vi "FSC.vi"(0 "System no.":i32=1 min=1 step=1, 1 "Board":i32=1 min=1 max=5 step=1, 2 "Axis 1 to scan":string, 3 "Axis 2 to scan":string, 4 "Range axis 1":dbl=0.1 format="%.4f", 5 "error in":errorcluster, 6 "Treshold level":dbl=0.1 format="%.3f", 7 "Step size":dbl=0.05 format="%.4f", 9 "Range axis 2":dbl=0.1 format="%.4f", 10 "Use #7 polling?":bool, 11 "Timeout (s)":dbl=300.0 min=1.0 max=4.0 step=1.0 format="%.2f", 12 "Stop refnum":refnum<vi>) -> (14 "Scan successful?":bool, 19 "error out":errorcluster)   [LabVIEW 2026]
doc: "Performs a 2D scan in specified axes, waits until scan is ready using #7 polling (if checked) and indicates whether scan was successful or not. If Stop refnum or Local stop is TRUE, VI sends #24 and stops. For a square scan, Range axis 2 must be identical to Range axis 1, otherwise a rectangular scan is performed. Timeout is only valid if Use #7 polling is FALSE.\n\nC-880: Use #7 polling = TRUE\nC-887, F-206, M-8X0: Use #7 polling = FALSE, Range axis 2 must be identical with Range axis 1 (no rectangular scan implemented). For GCS syntax version = GCS 2.0 or higher (check with CSV?.vi. If CSV?.vi is not supported, syntax version is GCS 1.0), VI calls FSS? automatically to determine if scan was successful or not."
uses:
  Communication/Syntax.ctl
  Communication/Global1.vi
panel:
  in  "Local stop":bool
  # "Performs an 2D scan in specified axes, waits until scan is \nready (using #7 polling if checked) and indicates whether scan was\nsuccessful or not.  If Stop refnum or Local stop is TRUE, VI sends #24 \nand stops. For a square scan, \"Range axis 2\" must be identical to \n\"Range axis 1\", otherwise a rectangular scan is performed. \"Timeout\" \nis only valid if \"Use #7 polling\" is FALSE."
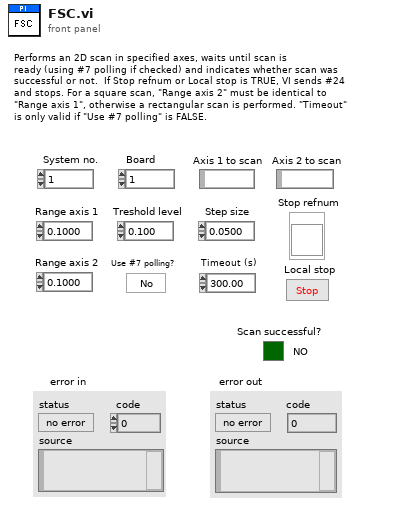
[diagram p1: front panel]
types:
  T1 = typedef "Syntax.ctl" = enum16{"GCS 1.0", "GCS 2.0", "GCS 3.0"}
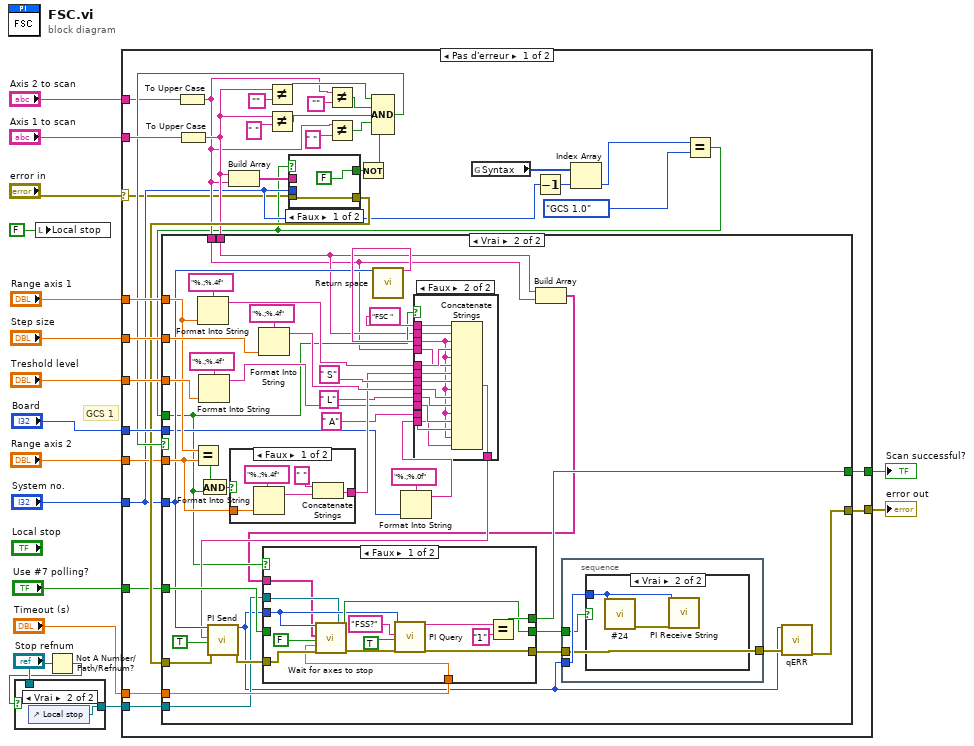
[diagram p0: block diagram]
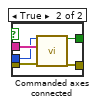
[diagram p3: hidden frame]
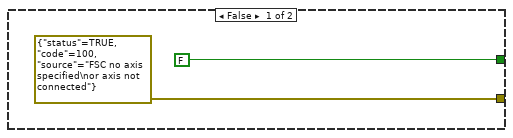
[diagram p4: hidden frame]
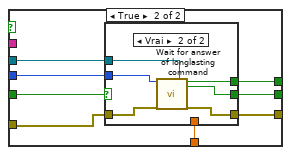
[diagram p5: hidden frame]
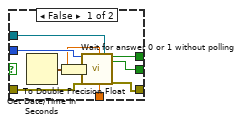
[diagram p6: hidden frame]
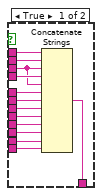
[diagram p7: hidden frame]
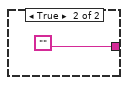
[diagram p9: hidden frame]
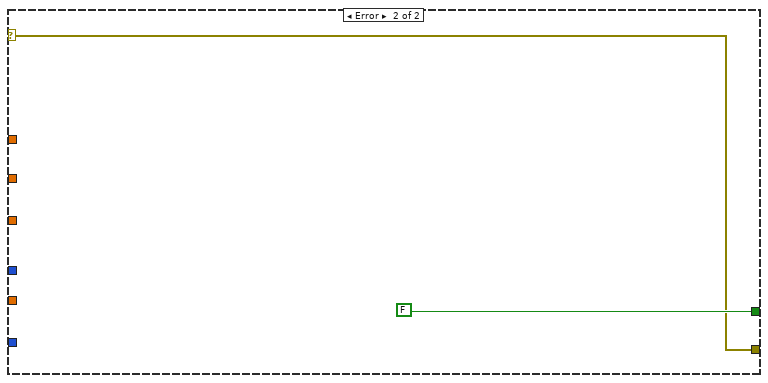
[diagram p10: hidden frame]
diagram:
  # "GCS 1"
  n1 = local write "Local stop"(FALSE ("Local stop")) -> ()
  n2 = Not A Number/Path/Refnum?(number/path/refnum="Stop refnum") -> (NaN/Path/Refnum?=w3:bool)
  n3 = case shown="Vrai" w3 {
    tunnel: [w18 w19] -> w2
    tunnel: "Stop refnum" -> [w18 _]
    frame False {
    }
    frame True {
      n4 = control-ref of="Local stop"() -> (w19:refnum<vi>)
    }
  }
  n5 = case shown="Pas d'erreur" "error in" {
    selector: "error in" -> [w21 w175]
    tunnel: "System no." -> [w23 _]
    tunnel: [w42 w175] -> w16
    tunnel: "Axis 1 to scan" -> [w53 _]
    tunnel: [w41 FALSE] -> w14
    tunnel: "Board" -> [w48 _]
    tunnel: "Range axis 1" -> [w47 _]
    tunnel: "Step size" -> [w46 _]
    tunnel: "Treshold level" -> [w45 _]
    tunnel: "Axis 2 to scan" -> [w37 _]
    tunnel: "Use #7 polling?" -> [w30 _]
    tunnel: "Timeout (s)" -> [w29 _]
    tunnel: "Range axis 2" -> [w28 _]
    tunnel: w2 -> [w27 _]
    frame No Error {
      n6 = To Upper Case(1:w37) -> (0:w31:string)
      n7 = To Upper Case(1:w53) -> (0:w32:string)
      n8 = Build Array(w32, w31) -> (w49:string[])
      n9 = Not Equal?(x=w32, y="") -> (x != y?=w50:bool)
      n10 = Not Equal?(x=w32, y=" ") -> (x != y?=w35:bool)
      n11 = Not Equal?(x=w31, y="") -> (x != y?=w34:bool)
      n12 = Not Equal?(x=w31, y=" ") -> (x != y?=w33:bool)
      n13 = global read "Global1.vi" "Syntax"() -> (w24:T1[])
      n14 = Decrement(x=w23) -> (x-1=w25:i32)
      n15 = Index Array(array=w24, index=w25) -> (element=w26:T1)
      n16 = Equal?(x=w26, y=Syntax."GCS 1.0") -> (x = y?=w22:bool)
      n17 = case shown="Faux" w22 {
        tunnel: w49 -> [_ w60]
        tunnel: w21 -> [w54 w59]
        tunnel: [w54 w58] -> w43
        tunnel: [FALSE ("Controller error") w57] -> w40
        tunnel: w23 -> [_ w56]
        frame False {
        }
        frame True {
          n18 = call "Commanded axes connected.vi"("System no."=w56, "Commanded axes"=w60, "error in"=w59) -> ("Controller error"=w57:bool, "error out"=w58:errorcluster)  [unwired: 15 out]
        }
      }
      n19 = Not(x=w40) -> (.not. x?=w39:bool)
      n20 = Compound Arithmetic op=AND(w50, w34, w35, w33, w39) -> (w44:bool)
      n21 = case shown="Vrai" w44 {
        tunnel: w48 -> [_ w69]
        tunnel: w47 -> [_ w87]
        tunnel: w46 -> [_ w93]
        tunnel: w32 -> [_ w65]
        tunnel: w45 -> [_ w95]
        tunnel: w43 -> [_ w100]
        tunnel: w23 -> [_ w74]
        tunnel: [errorcluster {"status"=TRUE, "code"=100, "source"="FSC no axis specified\nor axis not connected"} ("error out") w81] -> w42
        tunnel: [FALSE w80] -> w41
        tunnel: w31 -> [_ w64]
        tunnel: w30 -> [_ w91]
        tunnel: w29 -> [_ w90]
        tunnel: w28 -> [_ w86]
        tunnel: w27 -> [_ w77]
        tunnel: w22 -> [_ w66]
        frame False {
        }
        frame True {
          n22 = Equal?(x=w87, y=w86) -> (x = y?=w73:bool)
          n23 = Format Into String(format string="%.;%.4f" ("Format String"), w87) -> (resulting string=w92:string)  [unwired: 2 in, 1 out]
          n24 = Format Into String(format string="%.;%.4f" ("Format String"), w95) -> (resulting string=w83:string)  [unwired: 2 in, 1 out]
          n25 = And(x=w73, y=w66) -> (x .and. y?=w72:bool)
          n26 = case shown="Faux" w72 {
            tunnel: w86 -> [w172 _]
            tunnel: [w169 ""] -> w85
            frame False {
              n27 = Format Into String(format string="%.;%.4f" ("Format String"), w172) -> (resulting string=w170:string)  [unwired: 2 in, 1 out]
              n28 = Concatenate Strings(" ", w170) -> (w169:string)
            }
            frame True {
            }
          }
          n29 = Format Into String(format string="%.;%.4f" ("Format String"), w93) -> (resulting string=w89:string)  [unwired: 2 in, 1 out]
          n30 = call "Return space.vi"("System no."=w74) -> ("String out"=w75:string)  [unwired: 1 in, 17 out]
          n31 = Format Into String(format string="%.;%.0f" ("Format String"), w69) -> (resulting string=w68:string)  [unwired: 2 in, 1 out]
          n32 = case shown="Faux" w66 {
            tunnel: [w150 w163] -> w67
            tunnel: w92 -> [w149 w156]
            tunnel: w89 -> [w148 w162]
            tunnel: " S" -> [w147 w161]
            tunnel: w85 -> [w146 w154]
            tunnel: " L" -> [w145 w160]
            tunnel: w83 -> [w144 w159]
            tunnel: "FSC " -> [w143 w158]
            tunnel: w65 -> [w142 w157]
            tunnel: w64 -> [w141 w155]
            tunnel: w75 -> [w140 w151]
            tunnel: " A" -> [w139 w153]
            tunnel: w68 -> [w138 w152]
            frame True {
              n33 = Concatenate Strings(w143, w142, w140, w141, w140, w149, w146, w147, w148, w145, w144, w139, w138) -> (w150:string)
            }
            frame False {
              n34 = Concatenate Strings(w158, w157, w151, w156, w151, w155, w154, w161, w151, w162, w160, w151, w159, w153, w151, w152) -> (w163:string)
            }
          }
          n35 = call "PI Send.vi"("System no."=w74, "String to send"=w67, "Attach termination char.?"=TRUE ("Attach Linefeed?"), "error in"=w100) -> ("error out"=w98:errorcluster)  [unwired: 2 in, 13 out]
          n36 = Build Array(w65, w64) -> (w63:string[])
          n37 = case shown="Faux" w66 {
            tunnel: w98 -> [w109 w122]
            tunnel: w91 -> [_ w121]
            tunnel: w90 -> [w104 w120]
            tunnel: [w108 w119] -> w80
            tunnel: [w102 w118] -> w79
            tunnel: [w107 w117] -> w78
            tunnel: w77 -> [w105 w116]
            tunnel: w74 -> [w106 w115]
            tunnel: w63 -> [w103 _]
            frame False {
              n38 = call "Wait for axes to stop.vi"("System no."=w106, "Axes to wait for"=w103, "With status bit polling?"=FALSE, "Timeout (s)"=w104, "error in"=w109, "Stop refnum"=w105) -> ("Stopped"=w107:bool, "error out"=w111:errorcluster)  [unwired: 1 in, 11 out]
              n39 = call "PI Query.vi"("System no."=w106, "String to send"="FSS?", "Attach termination char.?"=TRUE ("Attach Linefeed?"), "error in"=w111) -> ("String read"=w101:string, "error out"=w102:errorcluster)  [unwired: 3 in, 11 out]
              n40 = Equal?(x=w101, y="1") -> (x = y?=w108:bool)
            }
            frame True {
              n41 = case shown="Vrai" w121 {
                tunnel: w115 -> [w131 w137]
                tunnel: w122 -> [w130 w136]
                tunnel: [w129 w135] -> w118
                tunnel: [w128 w134] -> w119
                tunnel: w120 -> [w126 _]
                tunnel: [w124 w133] -> w117
                tunnel: w116 -> [w125 w132]
                frame False {
                  n42 = Get Date/Time In Seconds() -> (seconds since 1Jan1904=w123:timestamp)
                  n43 = To Double Precision Float(number=w123) -> (double precision float=w127:dbl)
                  n44 = call "Wait for answer 0 or 1 without polling.vi"("System no."=w131, "error in"=w130, "Start time"=w127, "Timeout (s)"=w126, "Stop refnum"=w125) -> ("Scan successful?"=w128:bool, "Stopped"=w124:bool, "error out"=w129:errorcluster)  [unwired: 12 out]
                }
                frame True {
                  n45 = call "Wait for answer of longlasting command.vi"("System no."=w137, "error in"=w136, "Stop refnum"=w132) -> ("Answer"=w134:bool, "Stopped"=w133:bool, "error out"=w135:errorcluster)  [unwired: 14 out]
                }
              }
            }
          }
          n46 = stacked-sequence {
            tunnel: w74 -> [w166]
            tunnel: w79 -> [w165]
            tunnel: [w165] -> w82
            tunnel: w78 -> [w164]
            frame #0 {
              n47 = case shown="Vrai" w164 {
                tunnel: w166 -> [_ w168]
                frame False {
                }
                frame True {
                  n48 = call "#24.vi"("System no."=w168) -> ("error out"=w167:errorcluster)  [unwired: 1 in, 17 out]
                  n49 = call "PI Receive String.vi"("System no."=w168, "error in"=w167) -> ()  [unwired: 1 in, 17 out]
                }
              }
            }
          }
          n50 = call "qERR.vi"("System no."=w74, "error in"=w82) -> ("error out"=w81:errorcluster)  [unwired: 17 out]
        }
      }
    }
    frame Error {
    }
  }
  "error out" <- w16
  "Scan successful?" <- w14
